vi "LEP_RV_Close.vi"   [LabVIEW 2011]
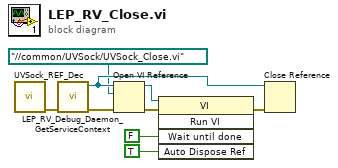
[diagram p0: block diagram]
diagram:
  n1 = call "UVSock_REF_Dec.vi"() -> ("error out"=w1:errorcluster)  [unwired: 1 in, 10 out]
  n2 = call "LEP_RV_Debug_Daemon_GetServiceContext.vi"("error in"=w1) -> ("error out"=w7:errorcluster, "service context"=w6:refnum<vi>)  [unwired: 9 out]
  n3 = Open VI Reference(application reference (local)=w6, vi path=path "../../common/UVSock/UVSock_Close.vi", error in (no error)=w7) -> (vi reference=w9:refnum<vi>, error out=w8:errorcluster)  [unwired: 3 out]
  n4 = invoke class="VI" method="Run VI"(reference=w9, error in=w8, "Wait until done"=FALSE ("Wait Until Done"), "Auto Dispose Ref"=TRUE ("Auto Dispose Reference")) -> (error out=w2:errorcluster)  [unwired: 1 in, 4 out]
  n5 = Close Reference(reference=w6, error in (no error)=w2) -> ()  [unwired: 1 out]
